vi "Actor Core.vi"(8 "error in":errorcluster, 11 "ConcreteModel in":refnum<class "ConcreteModel.lvclass">) -> (0 "error out":errorcluster, 3 "Actor out":refnum<class "Actor.lvclass">)   [LabVIEW 2017, in "Integration Test Launcher.lvlib" / "TopLevelApplication.lvlib" / "ConcreteModel.lvclass"]
doc: "(<B>Filename</B>: Actor Framework.lvlib:Actor.lvclass:Actor Core.vi)\n\nReceives messages to the actor, reacts to them, and initiates any error handling that may shut the actor down.\n\nDescendant classes may override this VI to append parallel tasks for the actor to complete while it handles messages. Overrides use the Call Parent Method node.\n\n<License>\nCopyright © 2020 Tymphany, LLC | All rights reserved\nwww.Tymphany.com\nHuijun <Huijun.Guo@Tymphany.com>\n</License>"
uses:
  <vilib>/gpm_packages/@cs/example/Integration Test/ConcreteModel/ConcreteModel.lvclass
  <vilib>/gpm_packages/@cs/example/Integration Test/Integration Test Launcher.lvlib
  <vilib>/gpm_packages/@cs/mva-core/Source/IModel/IModel/IModel.lvclass
  <vilib>/gpm_packages/@cs/mva-core/Source/RootModel/RootModel/RootModel.lvclass
  <vilib>/ActorFramework/Actor/Actor.lvclass
  C:/Program Files/National Instruments/LabVIEW 2017/vi.lib/gpm_packages/@cs/mva-core/Source/RootModel/RootModel/RootModel.lvclass
  C:/Program Files/National Instruments/LabVIEW 2017/vi.lib/gpm_packages/@cs/mva-core/Source/IModel/IModel/IModel.lvclass
  C:/Program Files/National Instruments/LabVIEW 2017/vi.lib/gpm_packages/@cs/mva-core/Source/IObserver/IObserver/IObserver.lvclass
  C:/Program Files/National Instruments/LabVIEW 2017/vi.lib/ActorFramework/Actor/Actor.lvclass
panel:
  in  "Process State":string
  in  "User Value (For Testing)":dbl=50.0 format="%#_13g"
  in  "Publish Period [ms]":u32=100
  in  "Stop Button":bool
  # "This Model Actor is only for a user to manipulate\nsome published data and observe the effect.\nThe Model is not seen in a real applcation."
  # "<-- Enter \"quad\" or \"chart\""
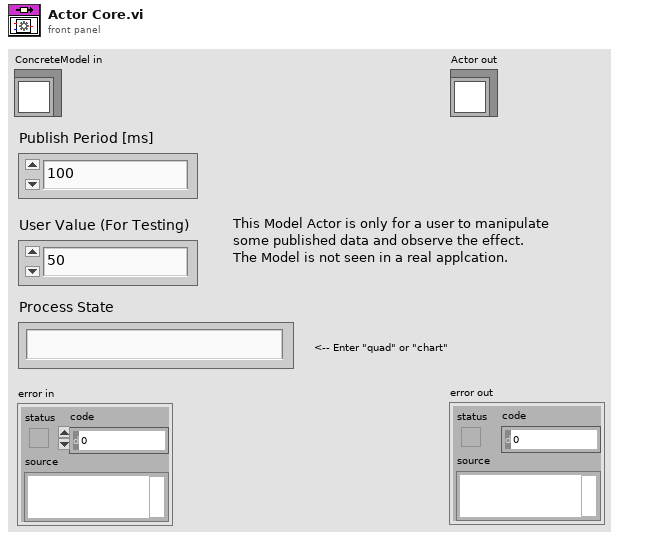
[diagram p1: front panel]
types:
  T1 = cluster{"seconds since 1Jan1904":timestamp, "number: 0 to 1":dbl}
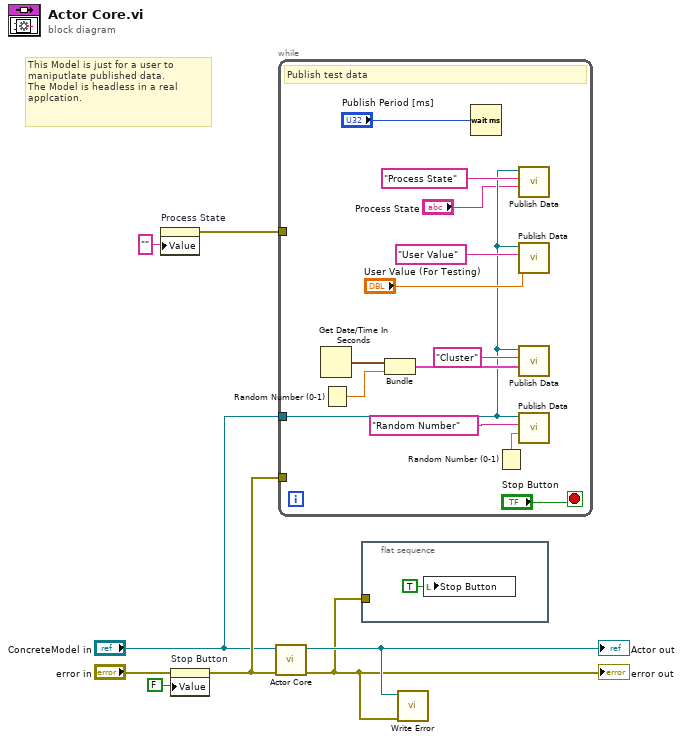
[diagram p0: block diagram]
diagram:
  # "This Model is just for a user to\nmaniputlate published data.\nThe Model is headless in a real\napplcation."
  n1 = property on="Process State" class="Str"("Value"="" ("Process State")) -> (error out=w4:errorcluster)  [unwired: 2 in, 1 out]
  n2 = property on="Stop Button" class="Bool (strict)"(error in="error in", "Value"=FALSE ("Stop Button")) -> (error out=w6:errorcluster)  [unwired: 1 in, 1 out]
  n3 = call-parent "Actor Core.vi"("error in"=w6, "Actor in"="ConcreteModel in") -> ("error out"=w1:errorcluster, "Actor out"=w2:refnum<class "Actor.lvclass">)  [unwired: 8 in]
  "error out" <- w1
  "Actor out" <- w2
  n4 = while {
    tunnel: w6 -> [_]
    tunnel: "ConcreteModel in" -> [w11]
    tunnel: w4 -> [_]
    stop <- "Stop Button" stop-if-true
    # "Publish test data"
    n5 = Get Date/Time In Seconds() -> (seconds since 1Jan1904=w17:timestamp)
    n6 = Random Number (0-1)() -> (number: 0 to 1=w18:dbl)
    n7 = Bundle("seconds since 1Jan1904"=w17, "number: 0 to 1"=w18) -> (w16:T1)  [unwired: 1 in]
    n8 = Wait (ms)(milliseconds to wait="Publish Period [ms]") -> ()  [unwired: 1 out]
    n9 = Random Number (0-1)() -> (number: 0 to 1=w9:dbl)
    n10 = call <vilib>:"Publish Data.vi"("Data to Publish"="Process State", "Datum Name"="Process State" ("Topic Name"), "IModel in"=w11) -> ()  [unwired: 7 in, 2 out]
    n11 = call <vilib>:"Publish Data.vi"("Data to Publish"="User Value (For Testing)", "Datum Name"="User Value" ("Topic Name"), "IModel in"=w11) -> ()  [unwired: 7 in, 2 out]
    n12 = call <vilib>:"Publish Data.vi"("Data to Publish"=w16, "Datum Name"="Cluster" ("Topic Name"), "IModel in"=w11) -> ()  [unwired: 7 in, 2 out]
    n13 = call <vilib>:"Publish Data.vi"("Data to Publish"=w9, "Datum Name"="Random Number" ("Topic Name"), "IModel in"=w11) -> ()  [unwired: 7 in, 2 out]
  }
  n14 = flat-sequence {
    tunnel: w1 -> [_]
    frame #0 {
      n15 = local write "Stop Button"(TRUE ("Stop Button")) -> ()
    }
  }
  n16 = call <vilib>:"Write Error.vi"("error in (no error)"=w1, "LabVIEW Object"=w2) -> ()  [unwired: 10 in]
